vi "Parse Graph Response.vi"(8 "error in":errorcluster, 11 "EF20 in":refnum<class "EF20.lvclass">) -> (0 "error out":errorcluster, 3 "EF20 out":refnum<class "EF20.lvclass">)   [LabVIEW 2018, in "EF20.lvlib" / "EF20.lvclass"]
uses:
  EF20.lvclass
  EF20.lvclass/EF20.ctl
  PPLs/Oven/Oven.lvlibp/Oven.lvclass
  C:/Projects/LabVIEW/PPLs/Oven/Oven.lvlibp/Oven.lvclass
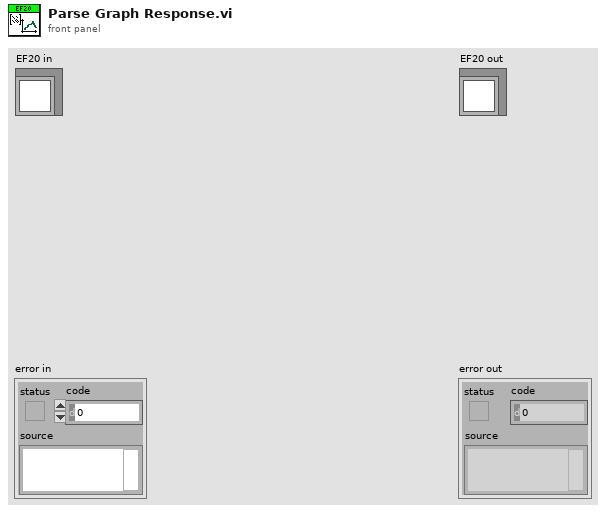
[diagram p1: front panel]
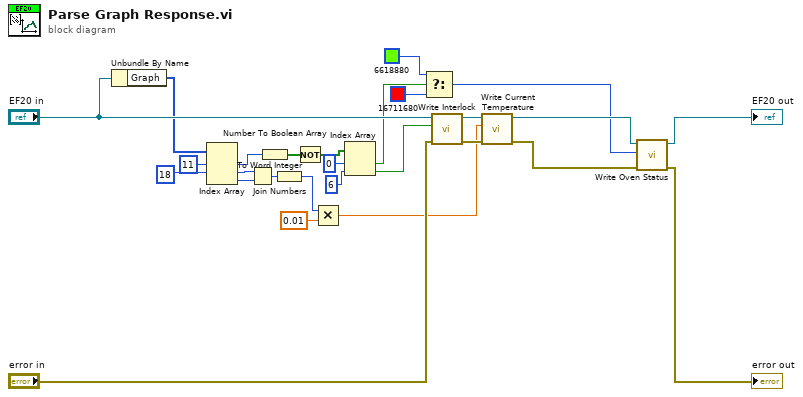
[diagram p0: block diagram]
diagram:
  n1 = Unbundle By Name("EF20 in") -> ("Graph"=w13:u8[])
  n2 = Index Array(array=w13, index #1=11 ("index"), index #2=18 ("index")) -> (element #1=w23:u8, element #2=w19:u8, element #3=w18:u8)  [unwired: 1 in]
  n3 = Join Numbers(hi=w19, lo=w18) -> ((hi.lo)=w17:u16)
  n4 = Number To Boolean Array(number=w23) -> (Boolean array=w24:bool[])
  n5 = To Word Integer(number=w17) -> (16bit integer=w15:i16)
  n6 = Not(x=w24) -> (.not. x?=w25:bool[])
  n7 = Multiply(x=w15, y=0.01) -> (x*y=w10:dbl)
  n8 = Index Array(array=w25, index #1=0 ("index"), index #2=6 ("index")) -> (element #1=w6:bool, element #2=w21:bool)
  n9 = Select(t=u32 6618880 ("Oven Status"), s=w6, f=u32 16711680 ("Oven Status")) -> (s? t:f=w3:u32)
  n10 = call "Write Interlock.vi"("error in (no error)"="error in", "Interlock"=w21, "Oven in"="EF20 in") -> ("error out"=w12:errorcluster, "Oven out"=w11:refnum<class "EF20.lvclass">)  [unwired: 7 in]
  n11 = call "Write Current Temperature.vi"("error in (no error)"=w12, "Current Temperature"=w10, "Oven in"=w11) -> ("error out"=w4:errorcluster, "Oven out"=w5:refnum<class "EF20.lvclass">)  [unwired: 7 in]
  n12 = call "Write Oven Status.vi"("error in (no error)"=w4, "Oven Status"=w3, "Oven in"=w5) -> ("error out"=→"error out":errorcluster, "Oven out"=→"EF20 out":refnum<class "EF20.lvclass">)  [unwired: 7 in]
